vi "binary_dataset_to_scaled_xyz.vi"(0 "binarySet":u8[](array[numeric]), 1 "measurementInterval":i32) -> (2 "x axis value":dbl, 3 "y axis value":dbl, 4 "z axis value":dbl)   [LabVIEW 2017]
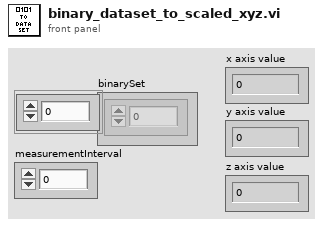
[diagram p1: front panel]
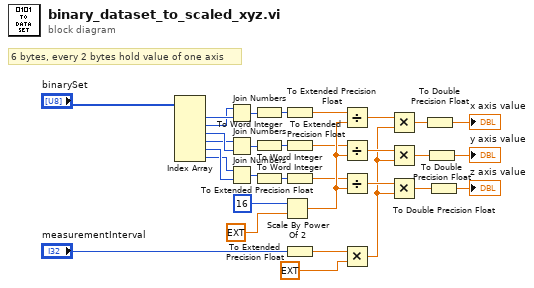
[diagram p0: block diagram]
diagram:
  # "6 bytes, every 2 bytes hold value of one axis"
  n1 = Index Array(array="binarySet") -> (element #1=w32:u8, element #2=w31:u8, element #3=w30:u8, element #4=w29:u8, element #5=w28:u8, element #6=w27:u8)  [unwired: 6 in]
  n2 = Join Numbers(hi=w31, lo=w32) -> ((hi.lo)=w26:u16)
  n3 = Join Numbers(hi=w29, lo=w30) -> ((hi.lo)=w25:u16)
  n4 = Join Numbers(hi=w27, lo=w28) -> ((hi.lo)=w24:u16)
  n5 = To Word Integer(number=w26) -> (16bit integer=w11:i16)
  n6 = To Word Integer(number=w25) -> (16bit integer=w12:i16)
  n7 = To Word Integer(number=w24) -> (16bit integer=w14:i16)
  n8 = Scale By Power Of 2(n=i16 16, x=ext 1.0) -> (x*2^n=w18:ext)
  n9 = To Extended Precision Float(1:w11) -> (0:w10:ext)
  n10 = To Extended Precision Float(1:w12) -> (0:w13:ext)
  n11 = To Extended Precision Float(1:w14) -> (0:w15:ext)
  n12 = To Extended Precision Float(1:"measurementInterval") -> (0:w9:ext)
  n13 = Divide(x=w10, y=w18) -> (x/y=w21:ext)
  n14 = Divide(x=w13, y=w18) -> (x/y=w20:ext)
  n15 = Divide(x=w15, y=w18) -> (x/y=w19:ext)
  n16 = Multiply(x=w9, y=ext 2.0) -> (x*y=w17:ext)
  n17 = Multiply(x=w21, y=w17) -> (x*y=w4:ext)
  n18 = Multiply(x=w20, y=w17) -> (x*y=w5:ext)
  n19 = Multiply(x=w19, y=w17) -> (x*y=w6:ext)
  n20 = To Double Precision Float(number=w4) -> (double precision float=→"x axis value":dbl)
  n21 = To Double Precision Float(number=w5) -> (double precision float=→"y axis value":dbl)
  n22 = To Double Precision Float(number=w6) -> (double precision float=→"z axis value":dbl)
